vi "opt_function_test2_thirdround.vi"(9 "output selector":T1={"objective function"=TRUE, "equality constraint"=TRUE, "inequality constraint"=TRUE}, 10 "data":variant, 11 "Initial parameters":dbl[](array[numeric])=[0.4703619837797438, 0.5159207753909103, -0.029460603986280604, -0.014620085820956148, -0.29884384559040056, 116.33878398505392, -107.90593243453512, 0.6430735689689421] step=1e-10 format="%#.33f") -> (0 "error out":errorcluster, 1 "Inequality Constraints":dbl[](array[numeric]), 2 "Equality Constraints":dbl[](array[numeric]), 3 "Global Error":dbl[](array[numeric])=[6.677242946482329])   [LabVIEW 2020]
uses:
  <vilib>/gmath/NumericalOptimization/cno_output select.ctl
  Camera software flag.vi
  Global line error.vi
  <vilib>/gmath/NI_Gmath.lvlib
panel:
  in  "Save input parameter history":path=path "C:/Users/Hannah/Downloads/input parameters"
  out "Global line error":dbl=6.677242946482329
  out "Numeric":i32=44046806
  out "Global line error 3":dbl=6.677242946482329
  in  "Acquisition time (ms)":dbl=76.0
  in  "Flyback time (ms)":dbl=24.0
  out "Waveform Graph 2":dbl[](graph)
  out "Global line error 2":dbl=14.137930338058743
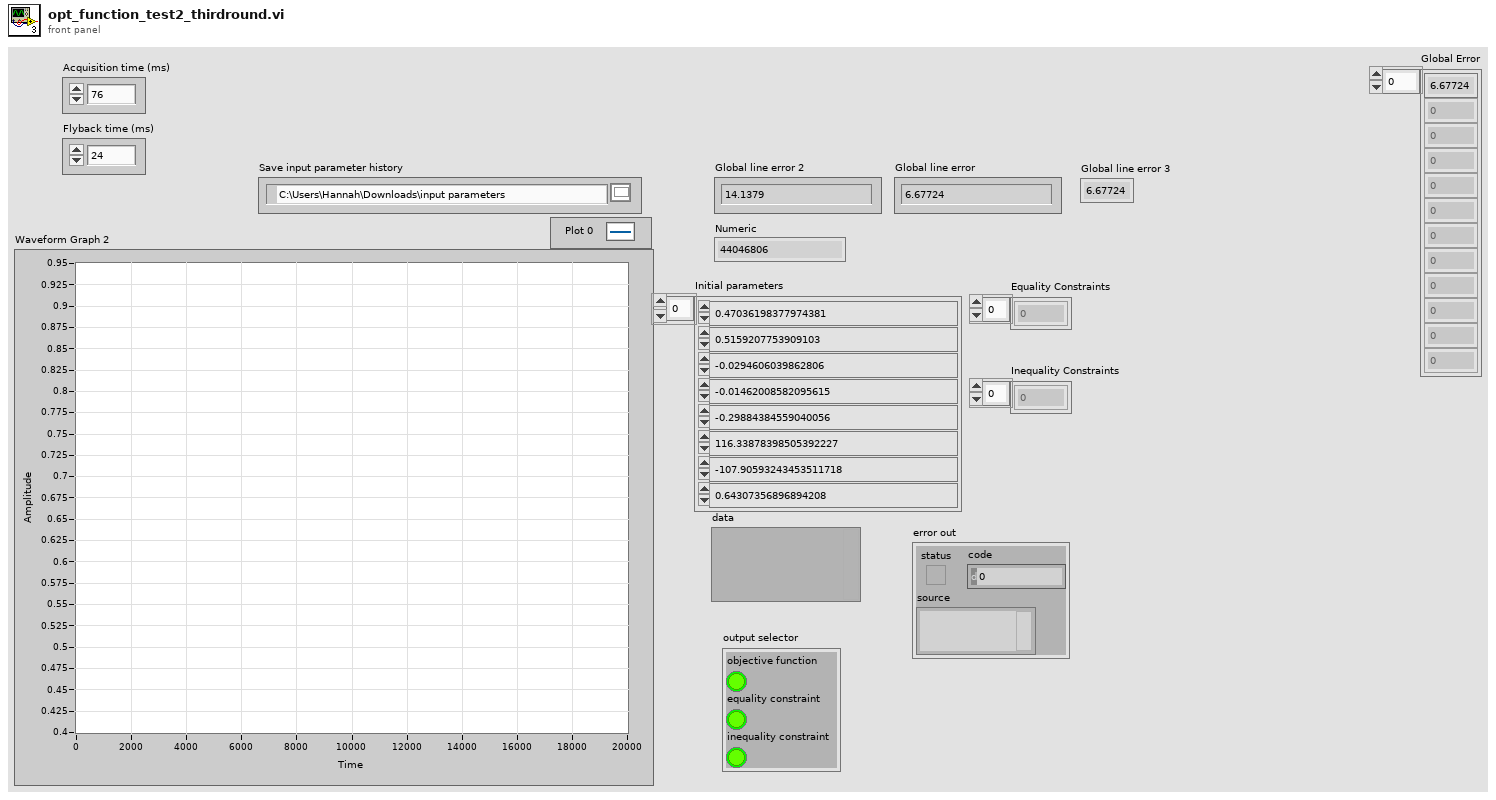
[diagram p1: front panel]
types:
  T1 = typedef "NI_Gmath.lvlib/cno_output select.ctl" = cluster{"objective function":bool, "equality constraint":bool, "inequality constraint":bool}
  T2 = enum16{"open", "replace", "create", "open or create", "replace or create", "replace or create with confirmation"}
  T3 = cluster{"Initial parameters[0]":dbl, "Initial parameters[1]":dbl, "Initial parameters[2]":dbl, "Initial parameters[3]":dbl, "Initial parameters[4]":dbl, "Initial parameters[5]":dbl, "Initial parameters[6]":dbl, "Initial parameters[7]":dbl, "Initial parameters[8]":dbl}
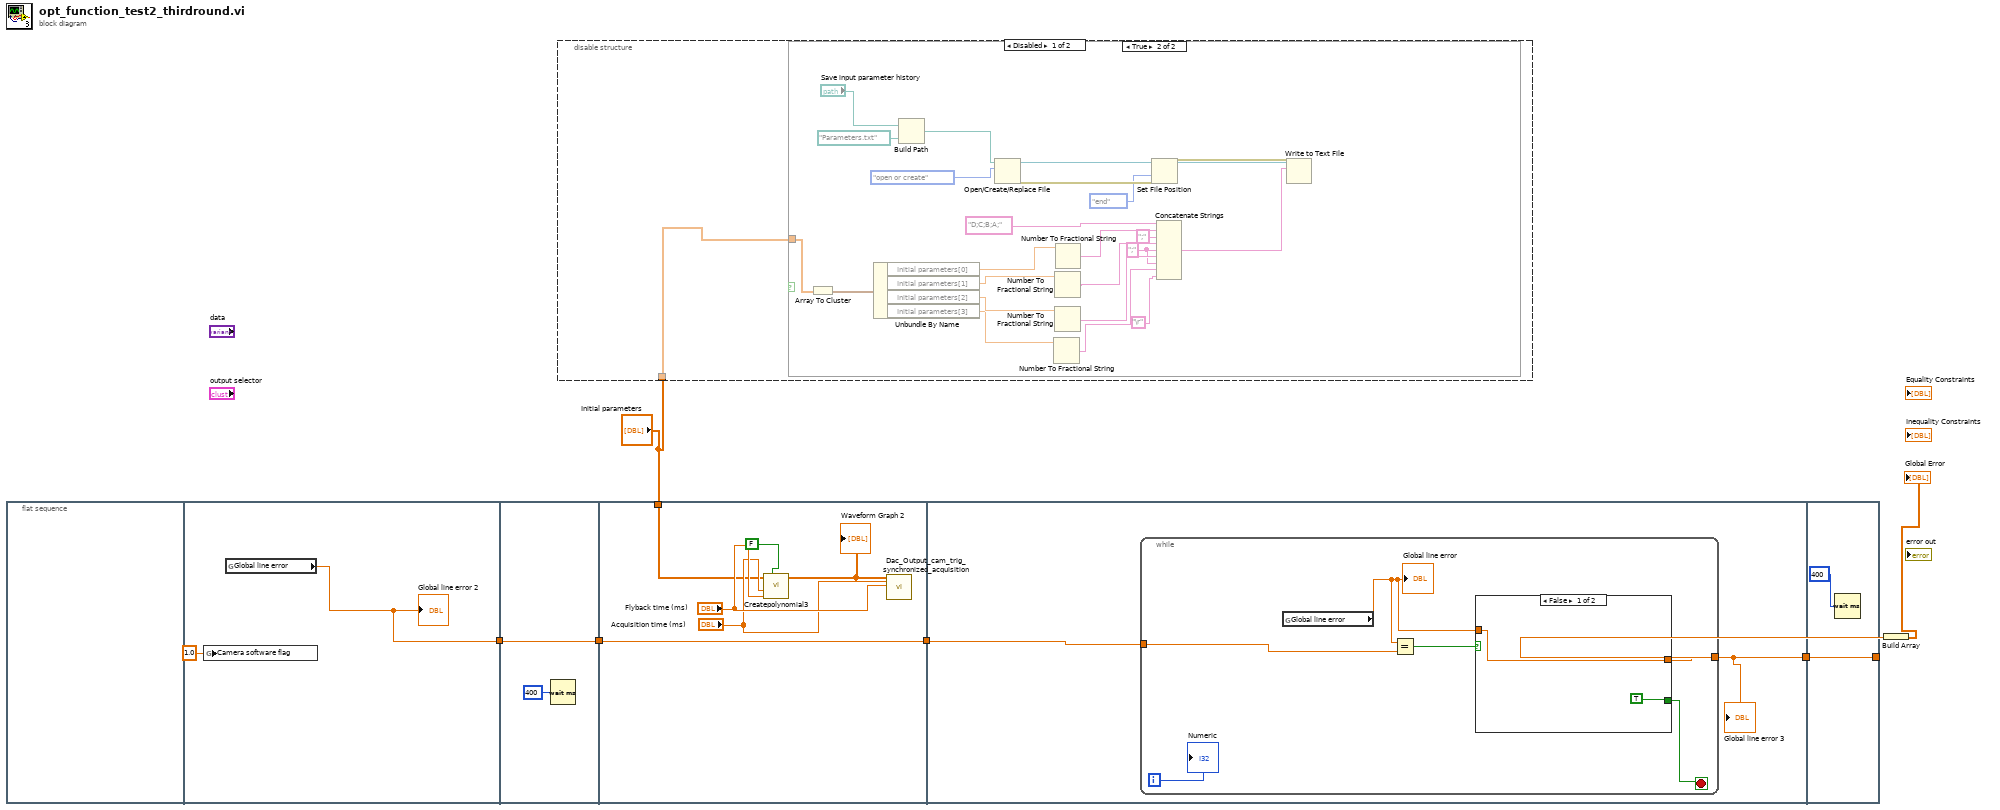
[diagram p0: block diagram]
diagram:
  n1 = flat-sequence {
    tunnel: [w9] -> w7
    tunnel: w7 -> [w11]
    tunnel: [w11] -> w6
    tunnel: w6 -> [w17]
    tunnel: [w17] -> w5
    tunnel: "Initial parameters" -> [w12]
    tunnel: w5 -> [w19]
    tunnel: [w18] -> w4
    tunnel: [w29] -> w2
    tunnel: w4 -> [w29]
    frame #0 {
    }
    frame #1 {
      n2 = global write "Camera software flag.vi" "Camera software flag"(1.0 ("Camera software flag")) -> ()
      n3 = global read "Global line error.vi" "Global line error"() -> (w9:dbl)
      "Global line error 2" <- w9
    }
    frame #2 {
      n4 = Wait (ms)(milliseconds to wait=u32 400) -> ()  [unwired: 1 out]
    }
    frame #3 {
      n5 = call "Createpolynomial3.vi"("Save calibration"=FALSE, "Flyback (ms)"="Flyback time (ms)", "Acquisition time (ms)"="Acquisition time (ms)", "P(x)"=w12) -> ("Generate two signals"=w13:dbl[])  [unwired: 7 in]
      "Waveform Graph 2" <- w13
      n6 = call "Dac_Output_cam_trig_synchronized_acquisition.vi"("Generate two signals"=w13, "Image acquisition time (ms)"="Acquisition time (ms)", "Delay between frames (ms)"="Flyback time (ms)") -> ()  [unwired: 17 in]
    }
    frame #4 {
      n7 = while {
        tunnel: w19 -> [w25]
        tunnel: [w22] -> w18
        i -> [w20]
        stop <- w21 stop-if-true
        n8 = global read "Global line error.vi" "Global line error"() -> (w23:dbl)
        "Global line error" <- w23
        n9 = Equal?(x=w23, y=w25) -> (x = y?=w24:bool)
        n10 = case shown="False" w24 {
          tunnel: w23 -> [w27 _]
          tunnel: [w27 _] -> w22
          tunnel: [TRUE _] -> w21
          frame False {
          }
          frame True {
          }
        }
        "Numeric" <- w20
      }
      "Global line error 3" <- w18
    }
    frame #5 {
      n11 = Wait (ms)(milliseconds to wait=u32 400) -> ()  [unwired: 1 out]
    }
  }
  n12 = disable-structure shown="Disabled" {
    disable-tunnel: "Initial parameters" -> [w30 _]
    frame Disabled {
      n13 = case shown="True" w31 {
        tunnel: w30 -> [_ w41]
        frame False {
        }
        frame True {
          w35 = ";" ("string")
          n14 = Array To Cluster(array=w41) -> (cluster=w40:T3)
          n15 = Unbundle By Name(w40) -> ("Initial parameters[0]"=w39:dbl, "Initial parameters[1]"=w38:dbl, "Initial parameters[2]"=w37:dbl, "Initial parameters[3]"=w34:dbl)
          n16 = Build Path(base path="Save input parameter history", name or relative path=path "Parameters.txt") -> (appended path=w55:path)
          n17 = Open/Create/Replace File(file path (use dialog)=w55, operation (0:open)=T2."open or create") -> (refnum out=w51:refnum<file>, error out=w52:errorcluster)  [unwired: 4 in, 1 out]
          n18 = Number To Fractional String(number=w34) -> (F-format string=w33:string)  [unwired: 3 in]
          n19 = Number To Fractional String(number=w38) -> (F-format string=w44:string)  [unwired: 3 in]
          n20 = Number To Fractional String(number=w37) -> (F-format string=w43:string)  [unwired: 3 in]
          n21 = Number To Fractional String(number=w39) -> (F-format string=w47:string)  [unwired: 3 in]
          n22 = Set File Position(refnum=w51, from (0:start)=enum16{"start", "end", "current"}."end", error in=w52) -> (refnum out=w53:refnum<file>, error out=w54:errorcluster)  [unwired: 1 in]
          n23 = Concatenate Strings("D;C;B;A;" ("text"), w47, ";" ("string"), w44, w35, w43, w35, w33, "\r") -> (w32:string)
          n24 = Write to Text File(file (use dialog)=w53, text=w32, error in=w54) -> ()  [unwired: 1 in, 3 out]
        }
      }
    }
    frame Enabled {
    }
  }
  n25 = Build Array(w2) -> (→"Global Error":dbl[])
